vi "SubStage_SetCellValue.vi"(0 "Row":i32, 1 "Col":i32, 2 "Value":string, 3 "error in (no error)":errorcluster, 4 "Excel._Worksheet":refnum<k7>) -> (5 "Excel._Worksheet":refnum<k7>, 6 "error out":errorcluster)   [LabVIEW 2015]
doc: "This VI sets the Value of the Cell in the WorkSheet designated by Row:Col to the input \"Value\". It first transforms the numeric row and column inputs to the Excel format of A1, B1 and so on. then it Executes the Range Method of the WorkSheet object and sets the \"Value\" property of the Range. It frees the automation Refnum of Range in each iteration of the loop."
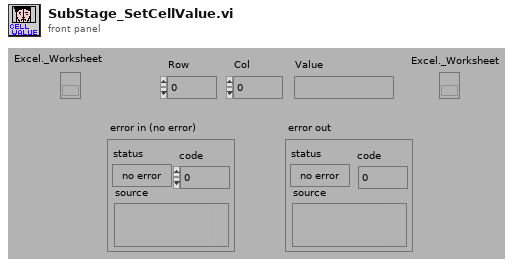
[diagram p1: front panel]
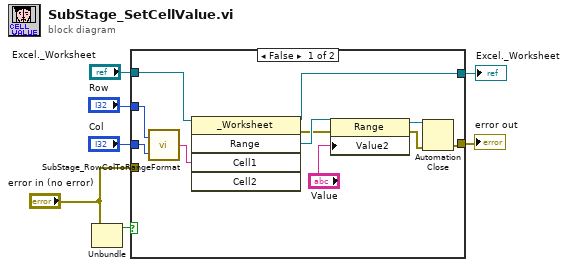
[diagram p0: block diagram]
diagram:
  n1 = Unbundle("error in (no error)") -> ("status"=w3:bool)  [unwired: 2 out]
  n2 = case shown="False" w3 {
    tunnel: "Col" -> [w10 _]
    tunnel: "Row" -> [w9 _]
    tunnel: "error in (no error)" -> [_ w20]
    tunnel: [w13 w20] -> w5
    tunnel: [w12 w19] -> w2
    tunnel: "Excel._Worksheet" -> [w11 w19]
    frame False {
      n3 = call "SubStage_RowColToRangeFormat.vi"("Column"=w10, "Row"=w9) -> ("Output String"=w8:string)
      n4 = invoke class="_Worksheet" method="Range"(reference=w11, "Cell1"=w8) -> (reference out=w12:refnum<k7>, error out=w17:errorcluster, "Range"=w18:refnum<k7>)  [unwired: 3 in, 2 out]
      n5 = property class="Range"(reference=w18, error in=w17, "Value2"="Value") -> (reference out=w15:refnum<k7>, error out=w14:errorcluster)
      n6 = Automation Close(3:w14, 5:w15) -> (0:w13:errorcluster)
    }
    frame True {
    }
  }
  "Excel._Worksheet" <- w2
  "error out" <- w5
